vi "parse_CMDStatus.vi"(8 "error in":errorcluster, 11 "msg in":string) -> (0 "error out":errorcluster, 2 "CMD Status":T1, 3 "msg out":string)   [LabVIEW 2018]
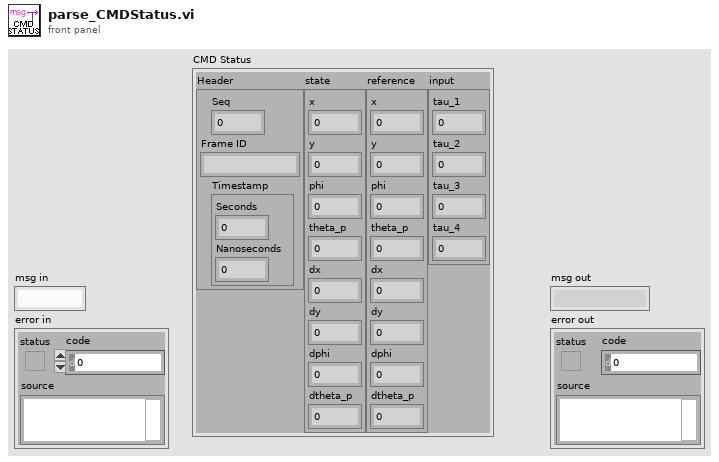
[diagram p1: front panel]
types:
  T1 = cluster{"Header":cluster{"Seq":u32, "Frame ID":string, "Timestamp":cluster{"Seconds":i32, "Nanoseconds":i32}}, "state":cluster{"x":dbl, "y":dbl, "phi":dbl, "theta_p":dbl, "dx":dbl, "dy":dbl, "dphi":dbl, "dtheta_p":dbl}, "reference":cluster{"x":dbl, "y":dbl, "phi":dbl, "theta_p":dbl, "dx":dbl, "dy":dbl, "dphi":dbl, "dtheta_p":dbl}, "input":cluster{"tau_1":dbl, "tau_2":dbl, "tau_3":dbl, "tau_4":dbl}}
  T2 = cluster{"Header":cluster{"Seq":u32, "Frame ID":string, "Timestamp":cluster{"Seconds":i32, "Nanoseconds":i32}}, "state":cluster{"x":dbl, "y":dbl, "phi":dbl, "theta_p":dbl, "dx":dbl, "dy":dbl, "dphi":dbl, "dtheta_p":dbl}, "reference":cluster{"x":dbl, "y":dbl, "phi":dbl, "theta_p":dbl, "dx":dbl, "dy":dbl, "dphi":dbl, "dtheta_p":dbl}, "input":cluster{"tau_1":dbl, "tau_2":dbl, "tau_3":dbl, "tau_4":dbl}, "feedforward":cluster{"tau_1":dbl, "tau_2":dbl, "tau_3":dbl, "tau_4":dbl}}
  T3 = cluster{"Seq":u32, "Frame ID":string, "Timestamp":cluster{"Seconds":i32, "Nanoseconds":i32}}
  T4 = cluster{"x":dbl, "y":dbl, "phi":dbl, "theta_p":dbl, "dx":dbl, "dy":dbl, "dphi":dbl, "dtheta_p":dbl}
  T5 = cluster{"tau_1":dbl, "tau_2":dbl, "tau_3":dbl, "tau_4":dbl}
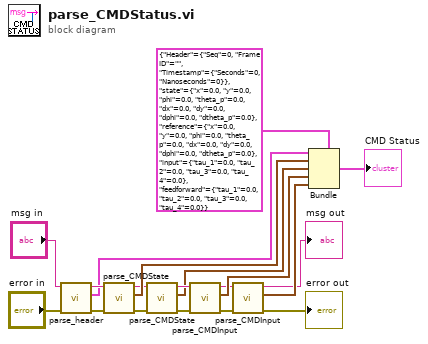
[diagram p0: block diagram]
diagram:
  n1 = call <userlib>:"parse_header.vi"("error in"="error in", "msg in"="msg in") -> ("error out"=w18:errorcluster, "Header"=w15:T3, "msg out"=w16:string)  [unwired: 3 in]
  n2 = call <userlib>:"parse_CMDState.vi"("error in"=w18, "msg in"=w16) -> ("error out"=w8:errorcluster, "CMD State"=w14:T4, "msg out"=w12:string)  [unwired: 7 in]
  n3 = call <userlib>:"parse_CMDState.vi"("error in"=w8, "msg in"=w12) -> ("error out"=w7:errorcluster, "CMD State"=w10:T4, "msg out"=w11:string)  [unwired: 7 in]
  n4 = call <userlib>:"parse_CMDInput.vi"("error in"=w7, "msg in"=w11) -> ("error out"=w5:errorcluster, "CMD Input"=w13:T5, "msg out"=w4:string)  [unwired: 7 in]
  n5 = call <userlib>:"parse_CMDInput.vi"("error in"=w5, "msg in"=w4) -> ("error out"=→"error out":errorcluster, "CMD Input"=w3:T5, "msg out"=→"msg out":string)  [unwired: 7 in]
  n6 = Bundle(cluster=T2 {"Header"={"Seq"=0, "Frame ID"="", "Timestamp"={"Seconds"=0, "Nanoseconds"=0}}, "state"={"x"=0.0, "y"=0.0, "phi"=0.0, "theta_p"=0.0, "dx"=0.0, "dy"=0.0, "dphi"=0.0, "dtheta_p"=0.0}, "reference"={"x"=0.0, "y"=0.0, "phi"=0.0, "theta_p"=0.0, "dx"=0.0, "dy"=0.0, "dphi"=0.0, "dtheta_p"=0.0}, "input"={"tau_1"=0.0, "tau_2"=0.0, "tau_3"=0.0, "tau_4"=0.0}, "feedforward"={"tau_1"=0.0, "tau_2"=0.0, "tau_3"=0.0, "tau_4"=0.0}}, "Header"=w15, "state"=w14, "reference"=w10, "input"=w13, "feedforward"=w3) -> (→"CMD Status":T2)
